vi "TestDAQ.vi"() -> ()   [LabVIEW 2018]
uses:
  DAQmx Read (Counter DBL 1Chan 1Samp).vi
  DAQmx Read (Counter U32 1Chan 1Samp).vi
  DAQmx Fill In Error Info.vi
panel:
  out "NeedleValveReadout":dbl format="%0.2f"
  out "Neutron Counts":u32
  in  "stop":bool
  out "Needle Valve Error":errorcluster
  out "Neutron Count Error":errorcluster
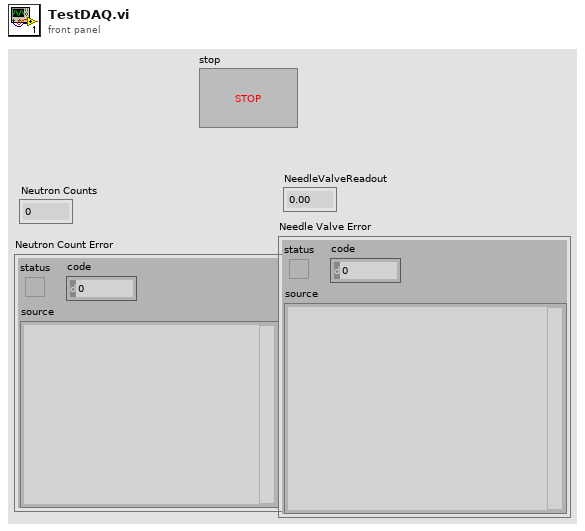
[diagram p1: front panel]
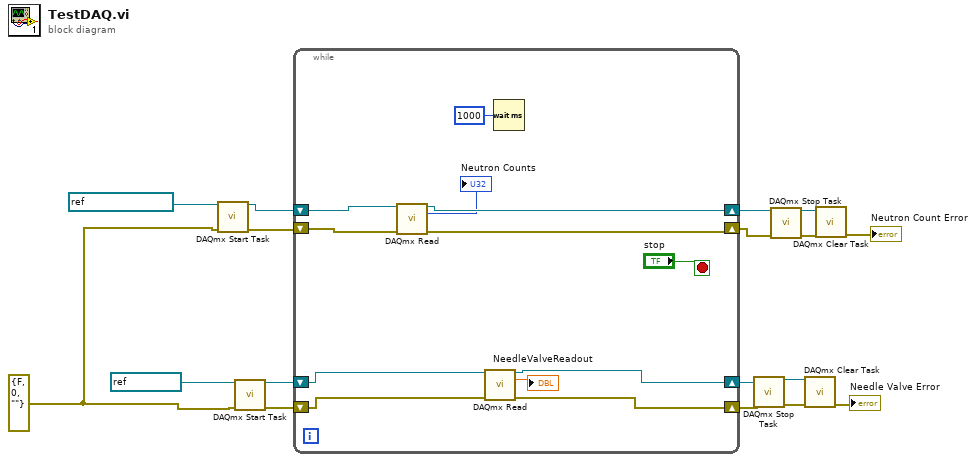
[diagram p0: block diagram]
diagram:
  w7 = errorcluster {"status"=FALSE, "code"=0, "source"=""} ("error in")
  n1 = call "DAQmx Start Task.vi"("task/channels in"=refnum<k21> "PencilDetector", "error in"=w7) -> ("task out"=w17:refnum<k21>, "error out"=w16:errorcluster)  [unwired: 12 in]
  n2 = call "DAQmx Start Task.vi"("task/channels in"=refnum<k21> "Encoder", "error in"=w7) -> ("task out"=w5:refnum<k21>, "error out"=w4:errorcluster)  [unwired: 12 in]
  n3 = while {
    shift-right: [w27] -> w15
    shift-left: w17 -> [w29]
    shift-right: [w26] -> w8
    shift-left: w16 -> [w28]
    shift-right: [w19] -> w3
    shift-left: w4 -> [w20]
    shift-right: [w18] -> w2
    shift-left: w5 -> [w21]
    stop <- "stop" stop-if-true
    n4 = call-poly "DAQmx Read.vi"("task/channels in"=w29, "error in"=w28) -> ("task out"=w27:refnum<k21>, "data"=→"Neutron Counts":u32, "error out"=w26:errorcluster)  [unwired: 11 in]
    n5 = call-poly "DAQmx Read.vi"("task/channels in"=w21, "error in"=w20) -> ("task out"=w18:refnum<k21>, "data"=→"NeedleValveReadout":dbl, "error out"=w19:errorcluster)  [unwired: 11 in]
    n6 = Wait (ms)(milliseconds to wait=u32 1000) -> ()  [unwired: 1 out]
  }
  n7 = call "DAQmx Stop Task.vi"("task/channels in"=w2, "error in"=w3) -> ("task out"=w14:refnum<k21>, "error out"=w13:errorcluster)  [unwired: 12 in]
  n8 = call "DAQmx Stop Task.vi"("task/channels in"=w15, "error in"=w8) -> ("task out"=w10:refnum<k21>, "error out"=w11:errorcluster)  [unwired: 12 in]
  n9 = call "DAQmx Clear Task.vi"("task in"=w14, "error in"=w13) -> ("error out"=→"Needle Valve Error":errorcluster)  [unwired: 13 in]
  n10 = call "DAQmx Clear Task.vi"("task in"=w10, "error in"=w11) -> ("error out"=→"Neutron Count Error":errorcluster)  [unwired: 13 in]
